vi "Get Metrics - PromTest1.vi"(7 "LabVIEW Web Service Request":refnum<class "Web Request.lvclass">, 11 "Registry":string="_default_registry") -> ()   [LabVIEW 2020]
uses:
  <vilib>/wsapi/Web Request.lvclass
  src/registry/session/Registry Session.lvclass
  src/metrics/metric/Metric.lvclass
panel:
  # "Use the Web Service Request input terminal to call the VIs on the Web Services palette. Do not remove it from the connector pane unless you don't need access to the palette."
  # "Each additional control wired to the connector pane will be available as an input in the URL. To include an indicator in terminal-mode output (the default setting), it must also be wired to the connector pane."
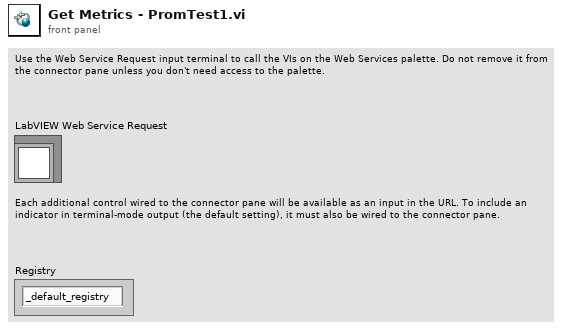
[diagram p1: front panel]
types:
  T1 = typedef "Registry.lvlib/Registry Session.lvclass/Session Handle.ctl" = refnum<data-value>
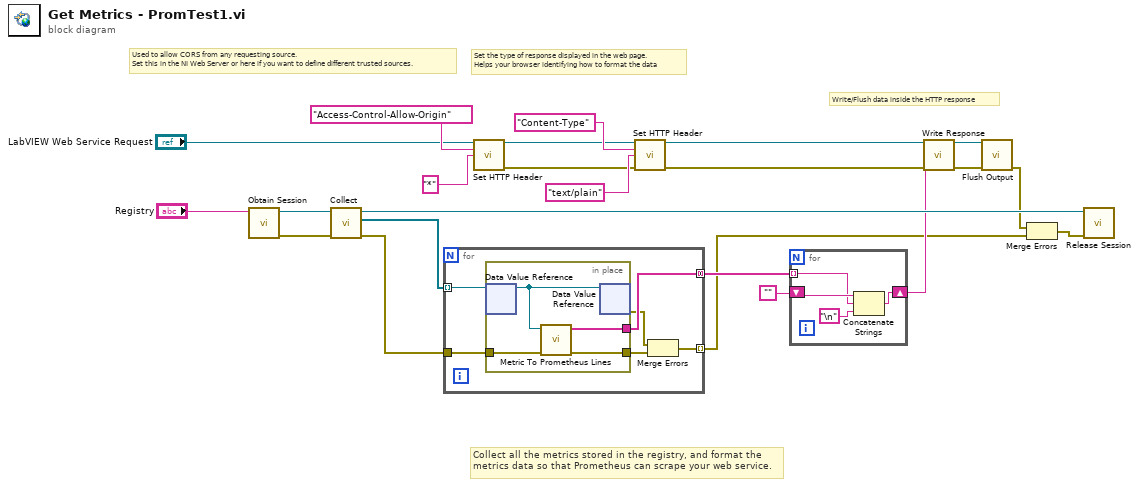
[diagram p0: block diagram]
diagram:
  # "Write/Flush data inside the HTTP response"
  # "Collect all the metrics stored in the registry, and format the metrics data so that Prometheus can scrape your web service."
  # "Set the type of response displayed in the web page.\nHelps your browser identifying how to format the data"
  # "Used to allow CORS from any requesting source.\nSet this in the NI Web Server or here if you want to define different trusted sources."
  n1 = call "Obtain Session.vi"("Session  Name ()"="Registry") -> ("error out"=w18:errorcluster, "Session Handle"=w19:T1)  [unwired: 9 in]
  n2 = call "Collect.vi"("error in (no error)"=w18, "Session Handle in"=w19) -> ("error out"=w1:errorcluster, "Metrics"=w2:refnum<data-value>[], "Session Handle out"=w17:T1)  [unwired: 7 in]
  n3 = for {
    tunnel: w2 -> [w29] mode=indexing
    tunnel: [w28] -> w4 mode=concatenating
    tunnel: w1 -> [w25]
    tunnel: [w24] -> w3 mode=indexing
    n4 = in-place {
      in-place-border: [w32] -> w28
      in-place-border: [w31] -> w26
      in-place-border: w25 -> [w30]
      n5 = in-place-dvr #1(w29) -> (w33:refnum<class "Metric.lvclass">)  [unwired: 1 out]
      n6 = call-dynamic "Metric To Prometheus Lines.vi"("error in (no error)"=w30, "Metrics.lvlib:Metric.lvclass"=w33) -> ("error out"=w31:errorcluster, "Prometheus Lines"=w32:string[])  [unwired: 8 in]
      n7 = in-place-dvr #1(w33) -> (w27:errorcluster)  [unwired: 1 out]
    }
    n8 = Merge Errors(w27, w26) -> (w24:errorcluster)
  }
  n9 = call <vilib>:"Set HTTP Header.vi"("LabVIEW Web Service Request"="LabVIEW Web Service Request", "header"="Access-Control-Allow-Origin", "header value"="*") -> ("LabVIEW Web Service Request out"=w13:refnum<class "Web Request.lvclass">, "error out"=w5:errorcluster)  [unwired: 11 in]
  n10 = call <vilib>:"Set HTTP Header.vi"("LabVIEW Web Service Request"=w13, "header"="Content-Type", "header value"="text/plain", "error in (no error)"=w5) -> ("LabVIEW Web Service Request out"=w12:refnum<class "Web Request.lvclass">, "error out"=w6:errorcluster)  [unwired: 10 in]
  n11 = for {
    tunnel: w4 -> [w35] mode=indexing
    shift-right: [w34] -> w8
    shift-left: "" -> [w37]
    n12 = Concatenate Strings(w37, w35, "\n") -> (w34:string)
  }
  n13 = call <vilib>:"Write Response.vi"("LabVIEW Web Service Request"=w12, "response string"=w8, "error in (no error)"=w6) -> ("LabVIEW Web Service Request out"=w16:refnum<class "Web Request.lvclass">, "error out"=w10:errorcluster)  [unwired: 11 in]
  n14 = call <vilib>:"Flush Output.vi"("LabVIEW Web Service Request"=w16, "error in (no error)"=w10) -> ("error out"=w7:errorcluster)  [unwired: 12 in, 1 out]
  n15 = Merge Errors(w7, w3) -> (w11:errorcluster)
  n16 = call "Release Session.vi"("error in (no error)"=w11, "Session Handle"=w17) -> ()  [unwired: 9 in, 1 out]
